vi "Initialize.vi"(8 "error in (no error)":errorcluster, 9 "DAQmx Digital Channel":tag, 10 "DAQmx Analog Channel":tag, 11 "UI in":refnum<class "UI.lvclass">) -> (0 "error out":errorcluster, 3 "UI out":refnum<class "UI.lvclass">)   [LabVIEW 2020, in "UI.lvlib" / "UI.lvclass"]
uses:
  UI.lvclass
  UI.lvclass/UI.ctl
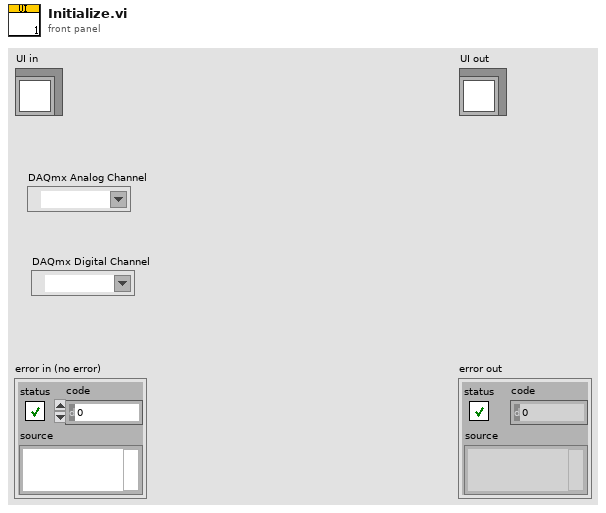
[diagram p1: front panel]
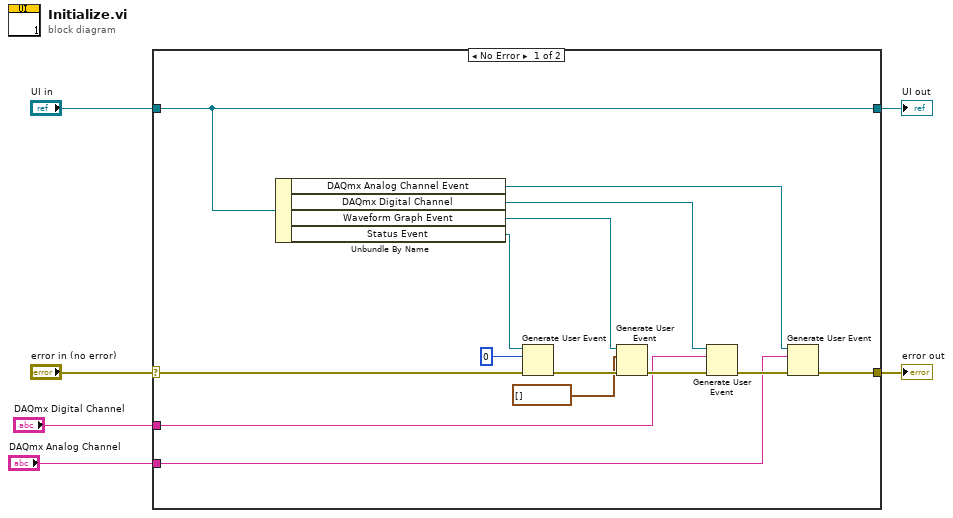
[diagram p0: block diagram]
diagram:
  n1 = case shown="No Error" "error in (no error)" {
    selector: "error in (no error)" -> [w18 w22]
    tunnel: [w10 w22] -> w5
    tunnel: [w20 w21] -> w3
    tunnel: "UI in" -> [w20 w21]
    tunnel: "DAQmx Digital Channel" -> [w8 _]
    tunnel: "DAQmx Analog Channel" -> [w7 _]
    frame No Error {
      n2 = Unbundle By Name(w20) -> ("DAQmx Analog Channel Event"=w9:refnum<user-event>, "DAQmx Digital Channel"=w12:refnum<user-event>, "Waveform Graph Event"=w15:refnum<user-event>, "Status Event"=w19:refnum<user-event>)
      n3 = Generate User Event(user event=w19, event data cluster=u8 0 ("event data"), error in=w18) -> (error out=w16:errorcluster)  [unwired: 1 in, 1 out]
      n4 = Generate User Event(user event=w15, event data cluster=waveform(dbl)[] [] ("event data"), error in=w16) -> (error out=w13:errorcluster)  [unwired: 1 in, 1 out]
      n5 = Generate User Event(user event=w12, event data cluster=w8, error in=w13) -> (error out=w11:errorcluster)  [unwired: 1 in, 1 out]
      n6 = Generate User Event(user event=w9, event data cluster=w7, error in=w11) -> (error out=w10:errorcluster)  [unwired: 1 in, 1 out]
    }
    frame Error {
    }
  }
  "error out" <- w5
  "UI out" <- w3
